vi "Read Num Nodes.vi"(8 "error in (no error)":errorcluster, 11 "abs_Composite in":refnum<class "bt_Composite.lvclass">) -> (0 "error out":errorcluster, 2 "Num Nodes":i32, 3 "abs_Composite out":refnum<class "bt_Composite.lvclass">)   [LabVIEW 2021, in "BT.lvlib" / "bt_Composite.lvclass"]
uses:
  bt_Composite.lvclass
  bt_Composite.lvclass/bt_Composite.ctl
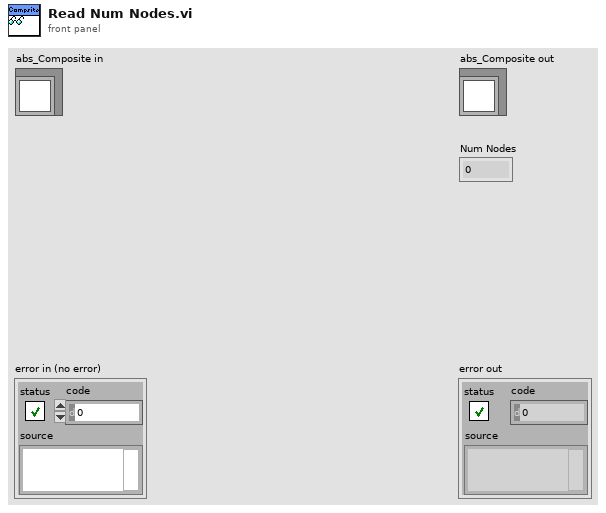
[diagram p1: front panel]
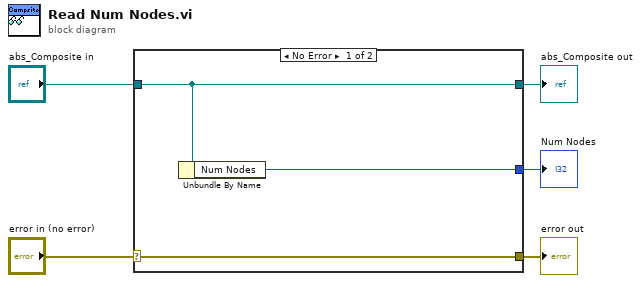
[diagram p0: block diagram]
diagram:
  n1 = case shown="No Error" "error in (no error)" {
    selector: "error in (no error)" -> [w8 w9]
    tunnel: [w8 w9] -> w4
    tunnel: [w7 w10] -> w2
    tunnel: "abs_Composite in" -> [w7 w10]
    tunnel: [w6 _] -> w1
    frame No Error {
      n2 = Unbundle By Name(w7) -> ("Num Nodes"=w6:i32)
    }
    frame Error {
    }
  }
  "error out" <- w4
  "abs_Composite out" <- w2
  "Num Nodes" <- w1
